vi "Uninstall All 1.0.vi"(7 "Restart Automatically (T)":bool=TRUE, 8 "error in (no error)":errorcluster, 11 "Session in":refnum<k21>) -> (0 "error out":errorcluster, 3 "Session out":refnum<k21>)   [LabVIEW 2017, in "nisyscfg.lvlib"]
uses:
  <vilib>/nisyscfg/nisyscfg.lvlib
  <vilib>/nisyscfg/Uninstall All.vi
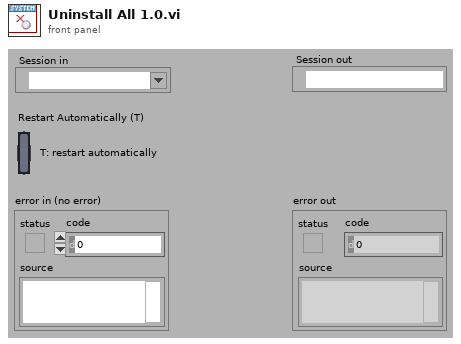
[diagram p1: front panel]
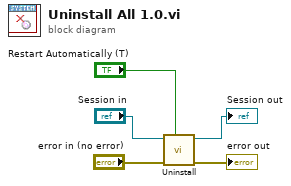
[diagram p0: block diagram]
diagram:
  n1 = call-poly <vilib>:"Uninstall.vi"("Restart Automatically (T)"="Restart Automatically (T)", "error in (no error)"="error in (no error)", "Session in"="Session in") -> ("error out"=→"error out":errorcluster, "Session out"=→"Session out":refnum<k21>)  [unwired: 7 in]
